vi "RefreshTimer.vi"(9 "Ticker Multiplier":dbl=10.0 format="%#_13g", 11 "Refresh Period [s]":dbl=5.0 format="%#_13g") -> (1 "Time to Next Refresh":dbl, 3 "Refresh Now?":bool)   [LabVIEW 2017, in "Client.lvlib" / "CommsServer.lvlib"]
uses:
  CommsServer.lvlib
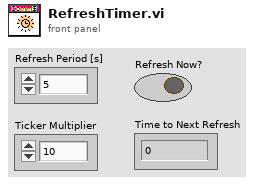
[diagram p1: front panel]
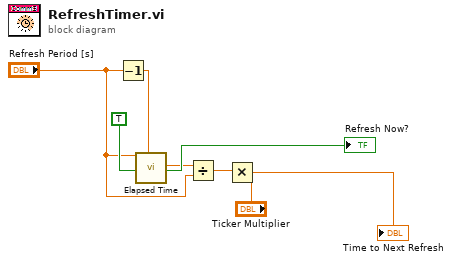
[diagram p0: block diagram]
diagram:
  n1 = Decrement(x="Refresh Period [s]") -> (x-1=w3:dbl)
  n2 = call "Elapsed Time"("Time Target (s)"="Refresh Period [s]", "Auto Reset"=TRUE, "Set Start Time (s)"=w3) -> ("Elapsed Time (s)"=w2:dbl, "Time has Elapsed"=→"Refresh Now?":bool)  [unwired: 9 in, 6 out]
  n3 = Divide(x=w2, y="Refresh Period [s]") -> (x/y=w1:dbl)
  n4 = Multiply(x=w1, y="Ticker Multiplier") -> (x*y=→"Time to Next Refresh":dbl)
